vi "Control Message Loop.vi"(8 "error in (no error)":errorcluster, 10 "DataQueuesAndNotifier":T1, 11 "Message Queues":T2) -> (0 "error out":errorcluster)   [LabVIEW 2019]
uses:
  support/Message Queue/All Message Queues.ctl
  support/Message Queue/Message Cluster.ctl
  DataQueuesAndNotifier.ctl
  Settings/System Running Settings.ctl
  HardwareAdapter/Support/Hardware Configuration.ctl
  HardwareAdapter/Support/Camera Configuration.ctl
  <vilib>/vision/Image Controls.llb/IMAQ Image.ctl
  Logging/Logging Configuration.ctl
  Controls/DeviceStatusCtl.ctl
  Controls/CallBack Refs.ctl
  Controls/Control Loop Status.ctl.ctl
  HardwareAdapter/Lasers/Laser Ctrl.ctl
  HardwareAdapter/Stages/Stage Ctrl.ctl
  support/Message Queue/Enqueue Message (Single).vi
  Global.vi
  <vilib>/Utility/error.llb/Error Cluster From Error Code.vi
  C:/RM21-MMicrosopeSource/HardwareAdapter/Camera/Dependencies/PVCamNET.dll
  HardwareAdapter/Camera/Dependencies/PVCamNET.dll
  C:/RM21-MMicrosopeSource/HardwareAdapter/Lasers/Dependencies/Oxxius_Boxx.dll
  HardwareAdapter/Lasers/Dependencies/Oxxius_Boxx.dll
  <vilib>/ErrorRing/Error Ring.xnode
  support/Message Queue/Message Queue.lvlib
  Acquisition.lvlib
  Logging/Logging.lvlib
  Settings/Settings.lvlib
panel:
  in  "Transfer XY":bool
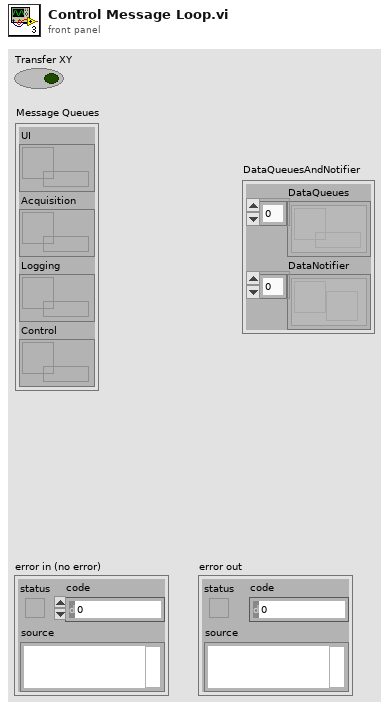
[diagram p1: front panel]
types:
  T1 = typedef "DataQueuesAndNotifier.ctl" = cluster{"DataQueues":refnum<queue>[], "DataNotifier":refnum<notifier>[]}
  T2 = typedef "Message Queue.lvlib/All Message Queues.ctl" = cluster{"UI":refnum<queue>, "Acquisition":refnum<queue>, "Logging":refnum<queue>, "Control":refnum<queue>}
  T3 = typedef "Settings.lvlib/System Running Settings.ctl" = cluster{"Hardware Configuration":T4, "Logging Configuration":T7, "HardWare Status":cluster{"CameraAndStages":T8, "Lasers":cluster{"IsConnected":cluster{"405":bool, "488":bool, "532":bool, "561":bool, "647":bool, "785":bool}, "IsOpened":cluster{"405":bool, "488":bool, "532":bool, "561":bool, "647":bool, "785":bool}}}, "CallBack Ref":T9}
  T4 = typedef "Hardware Configuration.ctl" = cluster{"Camera Configuration":T5, "Stages Configuration":cluster{"Resource":cluster{"NanoStage Ref":i32, "MicroStage Ref":i32, "TirfLock Ref":i32}, "SettingValues":cluster{"NanoState":cluster{"Time":dbl, "X":dbl, "Y":dbl, "Z":dbl}, "MicroState":cluster{"Time 2":dbl, "Z":dbl, "IsEPISet?":bool}, "TirfLock":cluster{"Time":dbl, "X":dbl, "Y":dbl, "Sum":dbl, "Calbrate":dbl, "LockedTarget":dbl, "Kp":dbl, "Ki":dbl, "Avg":dbl}}}, "Lasers Configuration":cluster{"SettingValues":cluster{"405 Power":sgl, "488 Power":sgl, "532 Power":sgl, "561 Power":sgl, "647 Power":sgl, "785 Power":sgl}, "Resource":cluster{"Library Ref":refnum<k24>, "Lasers Ref":cluster{"405 Ref":refnum<k24>, "488 Ref":refnum<k24>, "532 Ref":refnum<k24>, "561 Ref":refnum<k24>, "647 Ref":refnum<k24>, "785 Ref":refnum<k24>}}}}
  T5 = typedef "Camera Configuration.ctl" = cluster{"Setting":cluster{"Expouse":dbl, "Frames":dbl, "Interval":dbl}, "Resource":cluster{"CameraRef":refnum<k24>, "LibraryRef":refnum<k24>, "ImagesArray":T6[]}}
  T6 = typedef "IMAQ Image.ctl" = refnum<image>
  T7 = typedef "Logging.lvlib/Logging Configuration.ctl" = cluster{"Log File Base Folder":path, "FileSurfix":string, "TiffFileFullPath":path, "TimeStampFile Ref":refnum<file>, "NoteFileRef":refnum<file>, "HardWareInfoFileRef":refnum<file>, "QuickNoteInfo":string}
  T8 = typedef "DeviceStatusCtl.ctl" = cluster{"Camera":bool, "NanoStage":bool, "MicroStage":bool, "TIRFLock":bool}
  T9 = typedef "CallBack Refs.ctl" = cluster{"LiveAcq callback Ref":refnum<k27>, "AlbumAcq callback Ref":refnum<k27>, "SequenceAcq callback Ref":refnum<k27>, "Camera Status callback Ref":refnum<k27>}
  T10 = typedef "Control Loop Status.ctl.ctl" = enum16{"Idle", "Acquiring", "SequenceAcquire", "Tirf-Lock", "Lock XY", "Tirf-Lock,Lock XY", ""}
  T11 = typedef "Laser Ctrl.ctl" = cluster{"Laser Ref":refnum<k24>, "statue":bool, "Power":dbl, "Power Ref":refnum<vi>}
  T12 = typedef "Stage Ctrl.ctl" = cluster{"Axis":dbl, "value":dbl, "direction":bool}
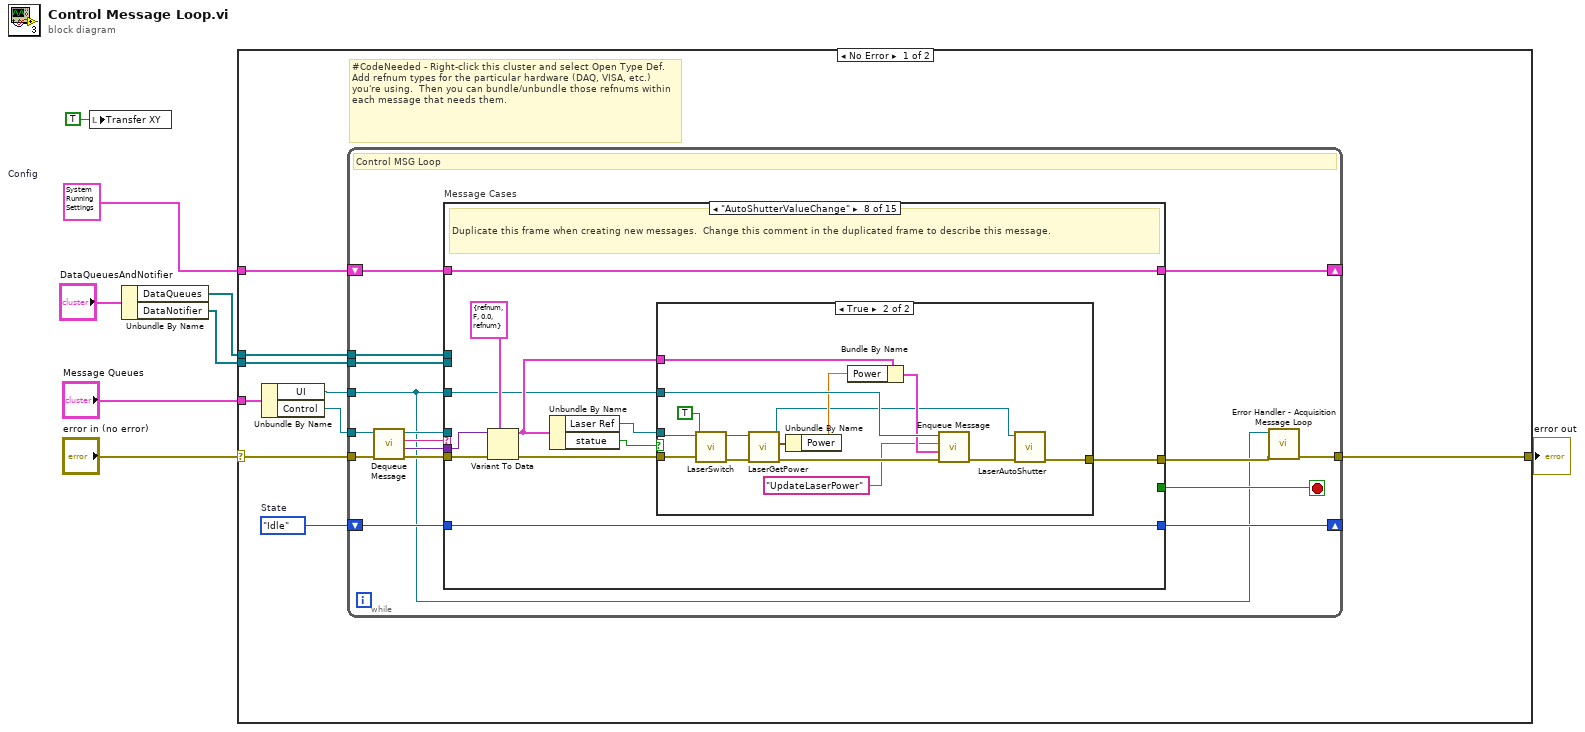
[diagram p0: block diagram]
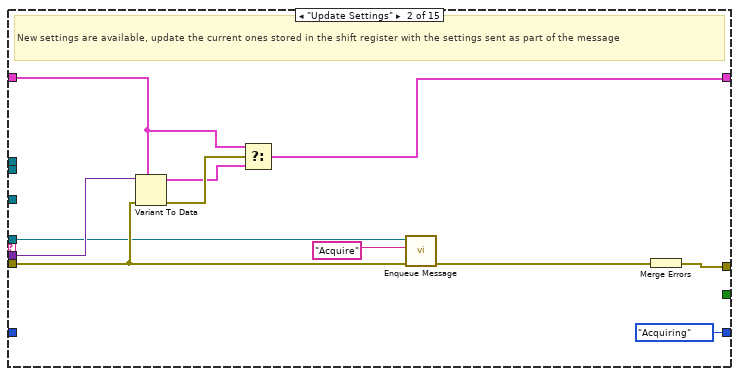
[diagram p3: hidden frame]
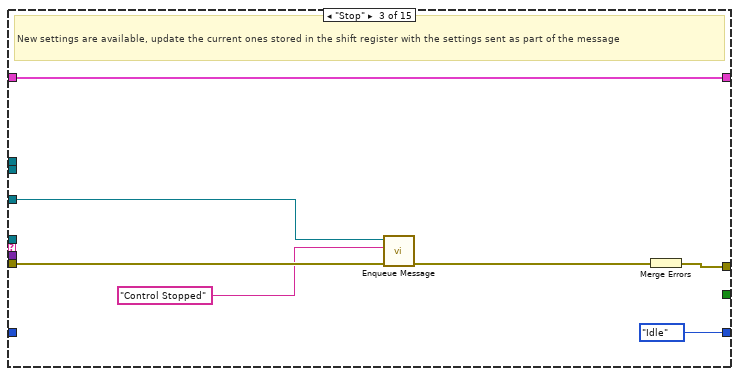
[diagram p4: hidden frame]
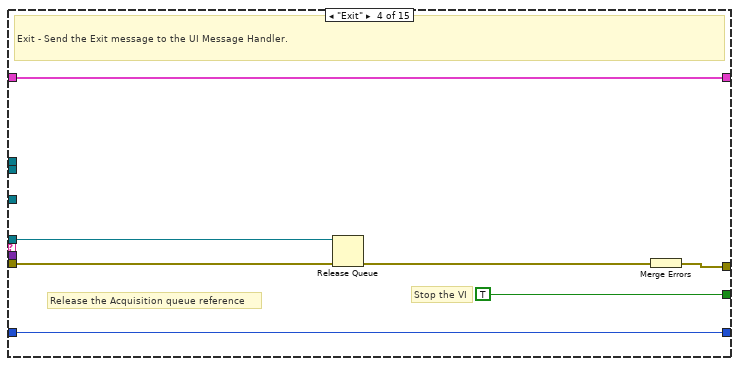
[diagram p5: hidden frame]
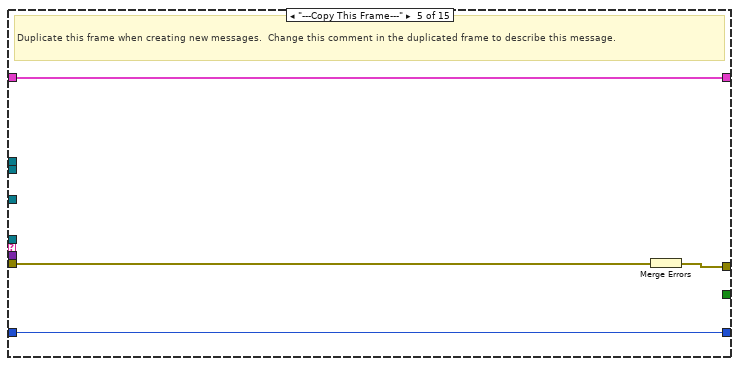
[diagram p6: hidden frame]
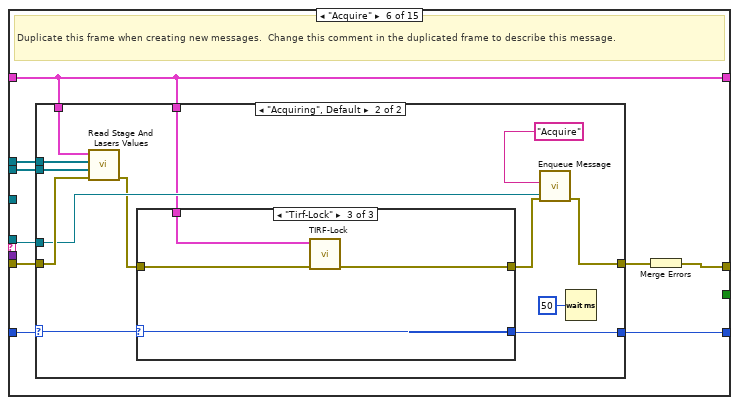
[diagram p7: hidden frame]
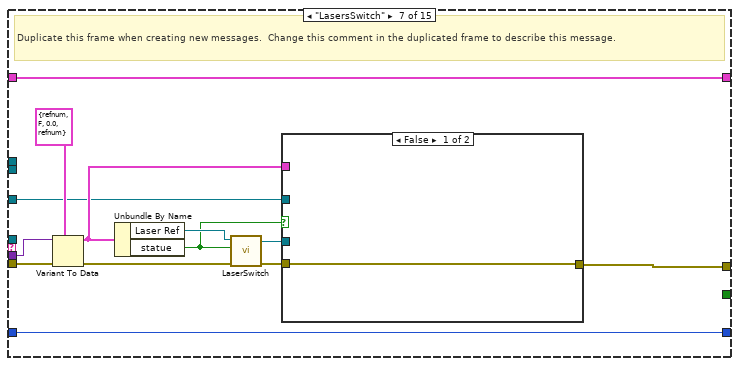
[diagram p11: hidden frame]
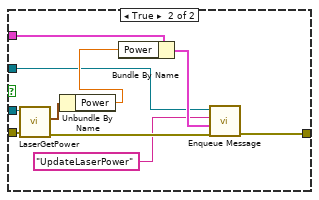
[diagram p12: hidden frame]
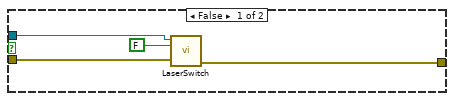
[diagram p13: hidden frame]
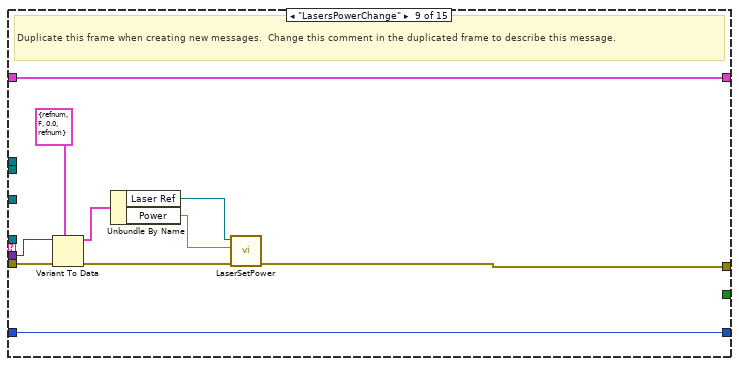
[diagram p14: hidden frame]
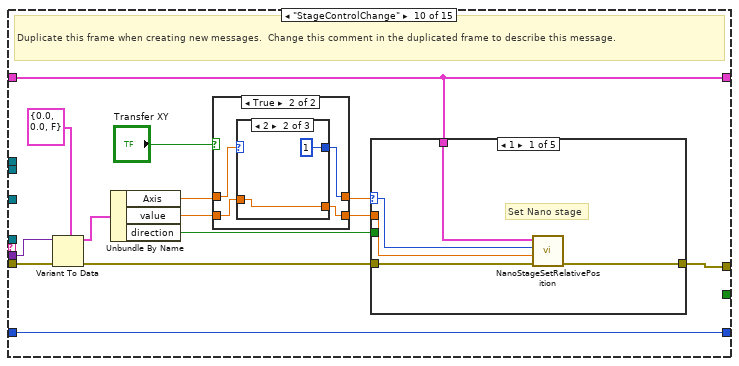
[diagram p15: hidden frame]
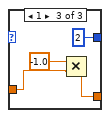
[diagram p18: hidden frame]
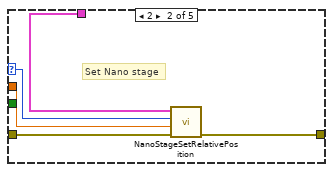
[diagram p19: hidden frame]
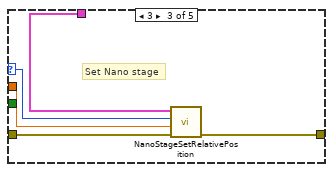
[diagram p20: hidden frame]
diagram:
  w5 = T3 {"Hardware Configuration"={"Camera Configuration"={"Setting"={"Expouse"=0.0, "Frames"=0.0, "Interval"=0.0}, "Resource"={"CameraRef"=refnum, "LibraryRef"=refnum, "ImagesArray"=[]}}, "Stages Configuration"={"Resource"={"NanoStage Ref"=0, "MicroStage Ref"=0, "TirfLock Ref"=0}, "SettingValues"={"NanoState"={"Time"=0.0, "X"=0.0, "Y"=0.0, "Z"=0.0}, "MicroState"={"Time 2"=0.0, "Z"=0.0, "IsEPISet?"=FALSE}, "TirfLock"={"Time"=0.0, "X"=0.0, "Y"=0.0, "Sum"=0.0, "Calbrate"=0.0, "LockedTarget"=0.0, "Kp"=0.0, "Ki"=0.0, "Avg"=0.0}}}, "Lasers Configuration"={"SettingValues"={"405 Power"=0.0, "488 Power"=0.0, "532 Power"=0.0, "561 Power"=0.0, "647 Power"=0.0, "785 Power"=0.0}, "Resource"={"Library Ref"=refnum, "Lasers Ref"={"405 Ref"=refnum, "488 Ref"=refnum, "532 Ref"=refnum, "561 Ref"=refnum, "647 Ref"=refnum, "785 Ref"=refnum}}}}, "Logging Configuration"={"Log File Base Folder"=path "", "FileSurfix"="", "TiffFileFullPath"=path "", "TimeStampFile Ref"=refnum, "NoteFileRef"=refnum, "HardWareInfoFileRef"=refnum, "QuickNoteInfo"=""}, "HardWare Status"={"CameraAndStages"={"Camera"=FALSE, "NanoStage"=FALSE, "MicroStage"=FALSE, "TIRFLock"=FALSE}, "Lasers"={"IsConnected"={"405"=FALSE, "488"=FALSE, "532"=FALSE, "561"=FALSE, "647"=FALSE, "785"=FALSE}, "IsOpened"={"405"=FALSE, "488"=FALSE, "532"=FALSE, "561"=FALSE, "647"=FALSE, "785"=FALSE}}}, "CallBack Ref"={"LiveAcq callback Ref"=refnum, "AlbumAcq callback Ref"=refnum, "SequenceAcq callback Ref"=refnum, "Camera Status callback Ref"=refnum}}  # Config
  n1 = local write "Transfer XY"(TRUE ("Transfer XY")) -> ()
  n2 = Unbundle By Name("DataQueuesAndNotifier") -> ("DataQueues"=w3:refnum<queue>[], "DataNotifier"=w2:refnum<notifier>[])
  n3 = case shown="No Error" "error in (no error)" {
    selector: "error in (no error)" -> [w14 w329]
    tunnel: "Message Queues" -> [w17 _]
    tunnel: [w15 w329] -> w7
    tunnel: w3 -> [w11 _]
    tunnel: w2 -> [w10 _]
    tunnel: w5 -> [w9 _]
    frame No Error {
      w12 = Control_Loop_Status.ctl."Idle"  # State
      # "#CodeNeeded - Right-click this cluster and select Open Type Def.  Add refnum types for the particular hardware (DAQ, VISA, etc.) you're using.  Then you can bundle/unbundle those refnums within each message that needs them."
      n4 = Unbundle By Name(w17) -> ("UI"=w13:refnum<queue>, "Control"=w16:refnum<queue>)
      n5 = while {
        tunnel: w16 -> [w26]
        shift-right: [w32] -> _
        shift-left: w9 -> [w33]
        tunnel: w13 -> [w20]
        shift-right: [w24] -> _
        shift-left: w12 -> [w25]
        tunnel: w14 -> [w30]
        tunnel: [w23] -> w15
        tunnel: w11 -> [w19]
        tunnel: w10 -> [w18]
        stop <- w31 stop-if-true
        # "Control MSG Loop"
        n6 = call "Dequeue Message.vi"("error in (no error)"=w30, "Message Queue"=w26) -> ("error out"=w29:errorcluster, "Message Data"=w27:variant, "Message"=w28:string, "dup Message Queue"=w21:refnum<queue>)  [unwired: 6 in]
        n7 = case "Message Cases" shown="\"AutoShutterValueChange\"" w28 {
          selector: w28 -> [_ _ _ _ _ _ _ _ _ _ _ _ _ _ w318]
          tunnel: w21 -> [_ w40 _ w59 _ w69 _ _ _ _ _ _ w230 _ _]
          tunnel: w29 -> [w36 w43 w52 w56 w65 w71 w108 w130 w159 w174 w216 w223 w237 w312 _]
          tunnel: [w36 w47 w54 w60 w63 w74 w99 w123 w156 w168 w214 w226 w239 w316 w319] -> w22
          tunnel: w33 -> [w35 w39 w53 w55 w64 w66 w110 w132 w161 w169 w218 w220 w229 w313 w321]
          tunnel: [w35 w44 w53 w55 w64 w66 w110 w132 w161 w169 w211 w221 w228 w313 w321] -> w32
          tunnel: [_ _ _ TRUE _ _ _ _ _ _ _ _ _ _ _] -> w31
          tunnel: w27 -> [_ w46 _ _ _ _ w107 w129 w158 w173 _ _ w235 _ _]
          tunnel: w20 -> [_ _ w50 _ _ _ w100 w126 _ _ w213 w225 w238 w315 _]
          tunnel: w25 -> [w34 _ _ w58 w62 w68 w109 w131 w160 w175 w219 w227 w232 w317 w320]
          tunnel: [w34 Control_Loop_Status.ctl."Acquiring" ("State") Control_Loop_Status.ctl."Idle" ("State") w58 w62 w67 w109 w131 w160 w175 w219 w227 w231 w317 w320] -> w24
          tunnel: w19 -> [_ _ _ _ _ w73 _ _ _ _ _ _ _ _ _]
          tunnel: w18 -> [_ _ _ _ _ w72 _ _ _ _ _ _ _ _ _]
          frame "Initialize" {
            # "Initialize  - Initialize is currently a no-op.  The hardware initialization takes place in the 'Start' message."
          }
          frame "Update Settings" {
            # "New settings are available, update the current ones stored in the shift register with the settings sent as part of the message"
            n8 = Variant To Data(error in=w43, type=w39, Variant=w46) -> (data=w38:T3, error out=w45:errorcluster)
            n9 = Select(t=w39, s=w45, f=w38) -> (s? t:f=w44:T3)
            n10 = call-poly "Enqueue Message.vi"("error in (no error)"=w43, "Message"="Acquire", "Message Queue"=w40) -> ("error out"=w42:errorcluster)  [unwired: 7 in, 1 out]
            n11 = Merge Errors(w42) -> (w47:errorcluster)
          }
          frame "Stop" {
            # "New settings are available, update the current ones stored in the shift register with the settings sent as part of the message"
            n12 = call-poly "Enqueue Message.vi"("error in (no error)"=w52, "Message"="Control Stopped", "Message Queue"=w50) -> ("error out"=w51:errorcluster)  [unwired: 7 in, 1 out]
            n13 = Merge Errors(w51) -> (w54:errorcluster)
          }
          frame "Exit" {
            # "Release the Acquisition queue reference"
            # "Stop the VI"
            # "Exit - Send the Exit message to the UI Message Handler."
            n14 = Release Queue(queue=w59, error in (no error)=w56) -> (error out=w57:errorcluster)  [unwired: 1 in, 2 out]
            n15 = Merge Errors(w57) -> (w60:errorcluster)
          }
          frame "---Copy This Frame---" {
            # "Duplicate this frame when creating new messages.  Change this comment in the duplicated frame to describe this message."
            n16 = Merge Errors(w65) -> (w63:errorcluster)
          }
          frame "Acquire" {
            # "Duplicate this frame when creating new messages.  Change this comment in the duplicated frame to describe this message."
            n17 = case shown="\"Acquiring\", Default" w68 {
              selector: w68 -> [w76 w81]
              tunnel: w66 -> [_ w89]
              tunnel: w73 -> [_ w88]
              tunnel: w72 -> [_ w87]
              tunnel: w71 -> [w75 w86]
              tunnel: [w75 w85] -> w70
              tunnel: w69 -> [_ w83]
              tunnel: [w76 w80] -> w67
              tunnel: w66 -> [_ w77]
              frame "Idle" {
              }
              frame "Acquiring", Default {
                n18 = call "Read Stage And Lasers Values.vi"("error in (no error)"=w86, "DataNotifier"=w87, "DataQueues"=w88, "Config In"=w89) -> ("error out"=w79:errorcluster)  [unwired: 7 in]
                n19 = case shown="\"Tirf-Lock\"" w81 {
                  selector: w81 -> [w91 w93 w97]
                  tunnel: [w91 w93 w97] -> w80
                  tunnel: w79 -> [w90 w92 w96]
                  tunnel: [w90 w92 w95] -> w78
                  tunnel: w77 -> [_ _ w94]
                  frame "Idle", Default {
                  }
                  frame "Acquiring" {
                  }
                  frame "Tirf-Lock" {
                    n20 = call "TIRF-Lock.vi"("error in (no error)"=w96, "Config"=w94) -> ("error Out"=w95:errorcluster)  [unwired: 8 in, 1 out]
                  }
                }
                n21 = call-poly "Enqueue Message.vi"("error in (no error)"=w78, "Message"="Acquire", "Message Queue"=w83) -> ("error out"=w85:errorcluster)  [unwired: 7 in, 1 out]
                n22 = Wait (ms)(milliseconds to wait=u32 50) -> ()  [unwired: 1 out]
              }
            }
            n23 = Merge Errors(w70) -> (w74:errorcluster)
          }
          frame "LasersSwitch" {
            # "Duplicate this frame when creating new messages.  Change this comment in the duplicated frame to describe this message."
            n24 = Variant To Data(error in=w108, type=T11 {"Laser Ref"=refnum, "statue"=FALSE, "Power"=0.0, "Power Ref"=refnum} ("Laser Ctrl"), Variant=w107) -> (data=w101:T11, error out=w106:errorcluster)
            n25 = Unbundle By Name(w101) -> ("Laser Ref"=w104:refnum<k24>, "statue"=w98:bool)
            n26 = call "LaserSwitch.vi"("error in (no error)"=w106, "SwitchON?"=w98, "reference In"=w104) -> ("error out"=w103:errorcluster, "reference out"=w102:refnum<k24>)  [unwired: 6 in]
            n27 = case shown="False" w98 {
              tunnel: w103 -> [w111 w121]
              tunnel: w102 -> [_ w120]
              tunnel: w101 -> [_ w118]
              tunnel: w100 -> [_ w113]
              tunnel: [w111 w112] -> w99
              frame False {
              }
              frame True {
                n28 = call "LaserGetPower.vi"("error in (no error)"=w121, "reference In"=w120) -> ("error out"=w119:errorcluster, "Power"=w117:cluster{"Time":dbl, "Power":dbl})  [unwired: 6 in, 1 out]
                n29 = Unbundle By Name(w117) -> ("Power"=w116:dbl)
                n30 = Bundle By Name(cluster=w118, "Power"=w116) -> (w115:T11)
                n31 = call-poly "Enqueue Message.vi"("error in (no error)"=w119, "Message Data"=w115, "Message"="UpdateLaserPower", "Message Queue"=w113) -> ("error out"=w112:errorcluster)  [unwired: 6 in, 1 out]
              }
            }
          }
          frame "AutoShutterValueChange" {
            # "Duplicate this frame when creating new messages.  Change this comment in the duplicated frame to describe this message."
            n32 = Variant To Data(error in=w130, type=T11 {"Laser Ref"=refnum, "statue"=FALSE, "Power"=0.0, "Power Ref"=refnum} ("Laser Ctrl"), Variant=w129) -> (data=w127:T11, error out=w125:errorcluster)
            n33 = Unbundle By Name(w127) -> ("Laser Ref"=w124:refnum<k24>, "statue"=w122:bool)
            n34 = case shown="True" w122 {
              tunnel: w127 -> [_ w151]
              tunnel: w126 -> [_ w150]
              tunnel: w125 -> [w135 w143]
              tunnel: w124 -> [w133 w137]
              tunnel: [w134 w140] -> w123
              frame False {
                n35 = call "LaserSwitch.vi"("error in (no error)"=w135, "SwitchON?"=FALSE, "reference In"=w133) -> ("error out"=w134:errorcluster)  [unwired: 6 in, 1 out]
              }
              frame True {
                n36 = call "LaserSwitch.vi"("error in (no error)"=w143, "SwitchON?"=TRUE, "reference In"=w137) -> ("error out"=w142:errorcluster, "reference out"=w138:refnum<k24>)  [unwired: 6 in]
                n37 = call "LaserGetPower.vi"("error in (no error)"=w142, "reference In"=w138) -> ("error out"=w149:errorcluster, "Power"=w148:cluster{"Time":dbl, "Power":dbl}, "reference out"=w139:refnum<k24>)  [unwired: 6 in]
                n38 = Unbundle By Name(w148) -> ("Power"=w147:dbl)
                n39 = Bundle By Name(cluster=w151, "Power"=w147) -> (w146:T11)
                n40 = call-poly "Enqueue Message.vi"("error in (no error)"=w149, "Message Data"=w146, "Message"="UpdateLaserPower", "Message Queue"=w150) -> ("error out"=w141:errorcluster)  [unwired: 6 in, 1 out]
                n41 = call "LaserAutoShutter.vi"("error in (no error)"=w141, "reference In"=w139) -> ("error out"=w140:errorcluster)  [unwired: 7 in, 1 out]
              }
            }
          }
          frame "LasersPowerChange" {
            # "Duplicate this frame when creating new messages.  Change this comment in the duplicated frame to describe this message."
            n42 = Variant To Data(error in=w159, type=T11 {"Laser Ref"=refnum, "statue"=FALSE, "Power"=0.0, "Power Ref"=refnum} ("Laser Ctrl"), Variant=w158) -> (data=w154:T11, error out=w157:errorcluster)
            n43 = Unbundle By Name(w154) -> ("Laser Ref"=w152:refnum<k24>, "Power"=w153:dbl)
            n44 = call "LaserSetPower.vi"("error in (no error)"=w157, "Power"=w153, "reference In"=w152) -> ("error out"=w156:errorcluster)  [unwired: 6 in, 1 out]
          }
          frame "StageControlChange" {
            # "Duplicate this frame when creating new messages.  Change this comment in the duplicated frame to describe this message."
            n45 = Variant To Data(error in=w174, type=T12 {"Axis"=0.0, "value"=0.0, "direction"=FALSE} ("Stage Ctrl"), Variant=w173) -> (data=w171:T12, error out=w170:errorcluster)
            n46 = Unbundle By Name(w171) -> ("Axis"=w165:dbl, "value"=w163:dbl, "direction"=w167:bool)
            n47 = case shown="True" "Transfer XY" {
              tunnel: w165 -> [w177 w181]
              tunnel: [w177 w180] -> w164
              tunnel: w163 -> [w176 w179]
              tunnel: [w176 w178] -> w162
              frame False {
              }
              frame True {
                n48 = case shown="2" w181 {
                  selector: w181 -> [w183 _ _]
                  tunnel: [w183 1 2] -> w180
                  tunnel: w179 -> [w182 w184 w187]
                  tunnel: [w182 w184 w188] -> w178
                  frame 0, Default {
                  }
                  frame 2 {
                  }
                  frame 1 {
                    n49 = Multiply(x=-1.0, y=w187) -> (x*y=w188:dbl)
                  }
                }
              }
            }
            n50 = case shown="1" w164 {
              selector: w164 -> [w193 w198 w203 _ _]
              tunnel: w170 -> [w194 w199 w204 w205 w210]
              tunnel: w162 -> [w192 w197 w202 _ w207]
              tunnel: w169 -> [w191 w196 w201 _ w206]
              tunnel: [w190 w195 w200 w205 w209] -> w168
              tunnel: w167 -> [_ _ _ _ w208]
              frame 1 {
                # "Set Nano stage"
                n51 = call "NanoStageSetRelativePosition.vi"("error in (no error)"=w194, "Increasement"=w192, "axis"=w193, "Config In"=w191) -> ("error out"=w190:errorcluster)  [unwired: 5 in, 1 out]
              }
              frame 2 {
                # "Set Nano stage"
                n52 = call "NanoStageSetRelativePosition.vi"("error in (no error)"=w199, "Increasement"=w197, "axis"=w198, "Config In"=w196) -> ("error out"=w195:errorcluster)  [unwired: 5 in, 1 out]
              }
              frame 3 {
                # "Set Nano stage"
                n53 = call "NanoStageSetRelativePosition.vi"("error in (no error)"=w204, "Increasement"=w202, "axis"=w203, "Config In"=w201) -> ("error out"=w200:errorcluster)  [unwired: 5 in, 1 out]
              }
              frame Default {
              }
              frame 4 {
                n54 = call "MicroStageSetRelativePosition.vi"("error in (no error)"=w210, "Move size (µm)"=w207, "Direction"=w208, "Config In"=w206) -> ("error out"=w209:errorcluster)  [unwired: 5 in, 1 out]
              }
            }
          }
          frame "TIRF-LockCalbrate" {
            # "Duplicate this frame when creating new messages.  Change this comment in the duplicated frame to describe this message."
            n55 = call "TIRF-LockCalbrate.vi"("error in (no error)"=w216, "QPD Axis"=TRUE, "Config"=w218) -> ("error out"=w215:errorcluster, "Config Out"=w211:T3)  [unwired: 7 in]
            n56 = call-poly "Enqueue Message.vi"("error in (no error)"=w215, "Message Data"=w211, "Message"="TIRF-LockCalbrate Finish", "Message Queue"=w213) -> ("error out"=w214:errorcluster)  [unwired: 6 in, 1 out]
          }
          frame "TIRF Find EPI" {
            # "Duplicate this frame when creating new messages.  Change this comment in the duplicated frame to describe this message."
            n57 = call "TIRF Find EPI.vi"("error in (no error)"=w223, "Config In"=w220) -> ("error out"=w222:errorcluster, "Config Out"=w221:T3)  [unwired: 8 in]
            n58 = call-poly "Enqueue Message.vi"("error in (no error)"=w222, "Message Data"=w221, "Message"="TIRF EPI Found", "Message Queue"=w225) -> ("error out"=w226:errorcluster)  [unwired: 6 in, 1 out]
          }
          frame "TIRF-Lock" {
            # "Duplicate this frame when creating new messages.  Change this comment in the duplicated frame to describe this message."
            n59 = Variant To Data(error in=w237, type=TRUE, Variant=w235) -> (data=w233:bool, error out=w236:errorcluster)
            n60 = case shown="True" w233 {
              tunnel: [w245 w271] -> w239
              tunnel: w238 -> [w244 w270]
              tunnel: w236 -> [w246 w272]
              tunnel: w232 -> [w243 w269]
              tunnel: [w242 w268] -> w231
              tunnel: w230 -> [w241 w267]
              tunnel: w229 -> [w240 w266]
              tunnel: [w240 w265] -> w228
              frame False {
                # "Tirf-Lock Stop"
                n61 = case shown="\"Tirf-Lock\"" w243 {
                  selector: w243 -> [_ _ w259]
                  tunnel: w246 -> [w250 w256 w262]
                  tunnel: [w247 w253 w260] -> w245
                  tunnel: w244 -> [w249 w255 w261]
                  tunnel: [Control_Loop_Status.ctl."Acquiring" ("State") Control_Loop_Status.ctl."Lock XY" ("State") w259] -> w242
                  tunnel: w241 -> [_ _ _]
                  frame "Tirf-Lock" {
                    n62 = call-poly "Enqueue Message.vi"("error in (no error)"=w250, "Message Data"="TIRF-Lock is Stop" ("Message"), "Message"="Update Status", "Message Queue"=w249) -> ("error out"=w247:errorcluster)  [unwired: 6 in, 1 out]
                  }
                  frame "Tirf-Lock,Lock XY" {
                    n63 = call-poly "Enqueue Message.vi"("error in (no error)"=w256, "Message Data"="TIRF-Lock is Stop" ("Message"), "Message"="Update Status", "Message Queue"=w255) -> ("error out"=w253:errorcluster)  [unwired: 6 in, 1 out]
                  }
                  frame "Idle", Default {
                    n64 = call-poly "Enqueue Message.vi"("error in (no error)"=w262, "Message Data"="TIRF-Lock is not running" ("Message"), "Message"="Update Status", "Message Queue"=w261) -> ("error out"=w260:errorcluster)  [unwired: 6 in, 1 out]
                  }
                }
              }
              frame True {
                # "Tirf-Locked Start"
                n65 = case shown="\"Idle\", Default" w269 {
                  selector: w269 -> [w274 _ _]
                  tunnel: w272 -> [w277 w290 w306]
                  tunnel: [w275 w291 w307] -> w271
                  tunnel: w270 -> [w276 w293 w309]
                  tunnel: [w274 Control_Loop_Status.ctl."Tirf-Lock,Lock XY" ("State") Control_Loop_Status.ctl."Tirf-Lock" ("State")] -> w268
                  tunnel: w267 -> [_ _ _]
                  tunnel: w266 -> [w273 w281 w298]
                  tunnel: [w273 w280 w296] -> w265
                  frame "Tirf-Lock", "Tirf-Lock,Lock XY" {
                    n66 = call-poly "Enqueue Message.vi"("error in (no error)"=w277, "Message Data"="TIRF-Lock is Running" ("Message"), "Message"="Update Status", "Message Queue"=w276) -> ("error out"=w275:errorcluster)  [unwired: 6 in, 1 out]
                  }
                  frame "Lock XY" {
                    n67 = Unbundle By Name(w281) -> ("Hardware Configuration.Stages Configuration.Resource.TirfLock Ref"=w285:i32)
                    n68 = call "Read_Tirf.vi"("Display"=TRUE, "Averages"=100, "Tirf-Handle"=w285) -> ("coerced(y)"=w282:dbl)  [unwired: 2 out]
                    n69 = call-poly "Enqueue Message.vi"("error in (no error)"=w290, "Message Data"="TIRF-Lock Start!" ("Message"), "Message"="Update Status", "Message Queue"=w293) -> ("error out"=w291:errorcluster)  [unwired: 6 in, 1 out]
                    n70 = Bundle By Name(cluster=w281, "Hardware Configuration.Stages Configuration.SettingValues.TirfLock.LockedTarget"=w282) -> (w280:T3)
                    n71 = global write "Global.vi" "TirfLockCounter"(0.0 ("TirfLockCounter")) -> ()
                    n72 = Initialize Array(0.0 ("Y"), 20 ("dimension size")) -> (w286:dbl[])
                    n73 = global write "Global.vi" "TirfLockPIDWindowArray"(w286) -> ()
                  }
                  frame "Idle", Default {
                    n74 = Unbundle By Name(w298) -> ("Hardware Configuration.Stages Configuration.Resource.TirfLock Ref"=w301:i32)
                    n75 = call "Read_Tirf.vi"("Display"=TRUE, "Averages"=100, "Tirf-Handle"=w301) -> ("coerced(y)"=w297:dbl)  [unwired: 2 out]
                    n76 = call-poly "Enqueue Message.vi"("error in (no error)"=w306, "Message Data"="TIRF-Lock Start!" ("Message"), "Message"="Update Status", "Message Queue"=w309) -> ("error out"=w307:errorcluster)  [unwired: 6 in, 1 out]
                    n77 = Bundle By Name(cluster=w298, "Hardware Configuration.Stages Configuration.SettingValues.TirfLock.LockedTarget"=w297) -> (w296:T3)
                    n78 = Initialize Array(0.0 ("Y"), 20 ("dimension size")) -> (w304:dbl[])
                    n79 = global write "Global.vi" "TirfLockPIDWindowArray"(w304) -> ()
                    n80 = global write "Global.vi" "TirfLockCounter"(0.0 ("TirfLockCounter")) -> ()
                  }
                }
              }
            }
          }
          frame "Lock XY" {
            # "Duplicate this frame when creating new messages.  Change this comment in the duplicated frame to describe this message."
            n81 = call-poly "Enqueue Message.vi"("error in (no error)"=w312, "Message"="TIRF-LockCalbrate Finish", "Message Queue"=w315) -> ("error out"=w316:errorcluster)  [unwired: 7 in, 1 out]
          }
          frame Default {
            # "'Default' case only runs if there is a message that isn't defined in any of the other cases.  Output a programming error."
            n82 = xnode "Error Ring"("parameter 0"=w318) -> ("error out"=w319:errorcluster)
          }
        }
        n83 = call "Error Handler - Acquisition Message Loop.vi"("error in (no error)"=w22, "Message Queue"=w20) -> ("dup error in"=w23:errorcluster)  [unwired: 8 in, 1 out]
      }
    }
    frame Error {
    }
  }
  "error out" <- w7
